vi "Init.vi"(8 "error in (no error)":errorcluster, 9 "Constant Action Data":string, 10 "HAL GOOP4.lvlib:Instrument Base":refnum<class "Instr Base.lvclass">, 11 "Virt Instrument Base in":refnum<class "Virt Instr Base.lvclass">) -> (0 "error out":errorcluster, 3 "Virt Instrument Base out":refnum<class "Virt Instr Base.lvclass">)   [LabVIEW 2023, in "HAL GOOP4.lvlib" / "Virt Instr Base.lvclass"]
uses:
  Virt Instr Base.lvclass
  Instrument Base/Instr Base.lvclass
  Virt Instr Base.lvclass/Virt Instr Base.ctl
  <vilib>/Utility/error.llb/Error Cluster From Error Code.vi
  <vilib>/ErrorRing/Error Ring.xnode
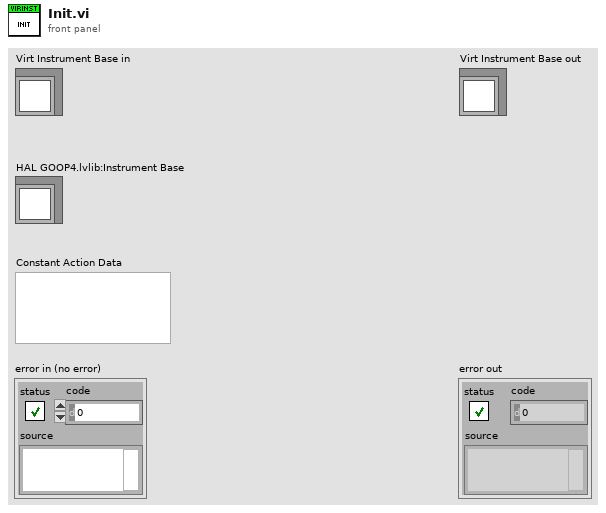
[diagram p1: front panel]
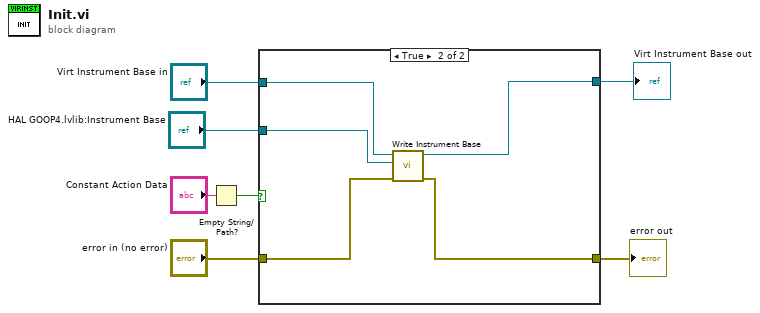
[diagram p0: block diagram]
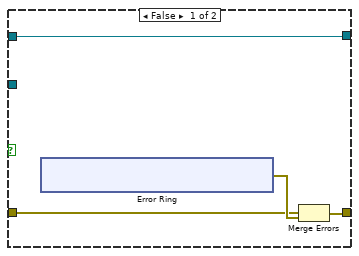
[diagram p2: hidden frame]
diagram:
  n1 = Empty String/Path?(string/path="Constant Action Data") -> (empty?=w1:bool)
  n2 = case shown="True" w1 {
    tunnel: "error in (no error)" -> [w9 w21]
    tunnel: [w11 w20] -> w6
    tunnel: "Virt Instrument Base in" -> [w8 w19]
    tunnel: [w8 w18] -> w4
    tunnel: "HAL GOOP4.lvlib:Instrument Base" -> [_ w17]
    frame False {
      n3 = xnode "Error Ring"() -> ("error out"=w10:errorcluster)
      n4 = Merge Errors(w9, w10) -> (w11:errorcluster)
    }
    frame True {
      n5 = call "Write Instrument Base.vi"("error in (no error)"=w21, "HAL GOOP4.lvlib:Instrument Base"=w17, "Virt Instrument Base in"=w19) -> ("error out"=w20:errorcluster, "Virt Instrument Base out"=w18:refnum<class "Virt Instr Base.lvclass">)  [unwired: 7 in]
    }
  }
  "error out" <- w6
  "Virt Instrument Base out" <- w4
